vi "FP calculate compass heading.vi"(1 "Y Location":dbl, 2 "X Location":dbl, 3 "Waypoint Y":dbl format="%#_13g", 4 "Waypoint X":dbl format="%#_13g") -> (0 "Heading":dbl)   [LabVIEW 2014]
doc: "This VI takes in the boat position and the desired waypoint and calculates a desired heading in the global corridinate system. It output the desired heading in degrees."
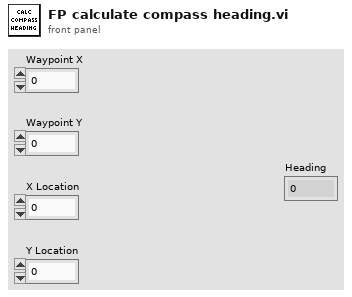
[diagram p1: front panel]
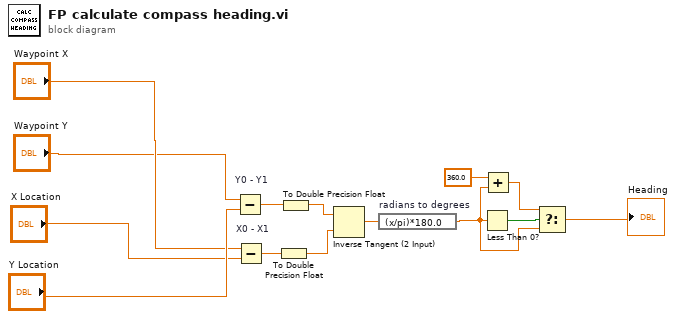
[diagram p0: block diagram]
diagram:
  n1 = Subtract "Y0 - Y1"(x="Waypoint Y", y="Y Location") -> (x-y=w8:dbl)
  n2 = Subtract "X0 - X1"(x="Waypoint X", y="X Location") -> (x-y=w9:dbl)
  n3 = To Double Precision Float(number=w9) -> (double precision float=w10:dbl)
  n4 = To Double Precision Float(number=w8) -> (double precision float=w11:dbl)
  n5 = Inverse Tangent (2 Input)(1:w10, 2:w11) -> (0:w12:dbl)
  n6 = expression code="(x/pi)*180.0" "radians to degrees"(w12) -> (w14:dbl)
  n7 = Less Than 0?(x=w14) -> (x < 0?=w13:bool)
  n8 = Add(x=360.0, y=w14) -> (x+y=w6:dbl)
  n9 = Select(t=w6, s=w13, f=w14) -> (s? t:f=→"Heading":dbl)
